vi "StateMachine V2.vi"() -> ()   [LabVIEW 2014]
uses:
  <vilib>/DAQmx/create/channels.llb/DAQmx Create Channel (AI-Voltage-Basic).vi
  <vilib>/DAQmx/configure/timing.llb/DAQmx Timing (Sample Clock).vi
  <vilib>/DAQmx/read.llb/DAQmx Read (Analog 1D Wfm NChan NSamp).vi
  <vilib>/Waveform/WDTOps.llb/WDT Index Channel DBL.vi
  <resource>/objmgr/daqmx.rc
panel:
  in  "Error In":errorcluster
  out "Final Data Array":dbl[][](array[numeric])
  in  "index":i32 caption="Index"
  out "Time & Y Array":dbl[][](array[numeric])
  out "Time Array":dbl[](array[numeric])
  out "Y Array":dbl[](array[numeric])
  out "Data Logging Done?":bool
  in  "Write Data in File":bool
  out "Recording ON time [ms]":u32
  out "Timer-Wert (ms)":u32
  in  "Timer [ms]":u32=2000
  out "Storing ON?":bool
  in  "Stopp":bool
  in  "Store Data in Array":bool
  out "State":T1(ring)
  out "Signalverlaufsgraph":waveform(dbl)[](graph)
  in  "samples per channel":i32=256 caption="Samples pro Kanal"
  out "SampleTakt.Rate":dbl
  in  "rate":dbl=2560.0 caption="Rate" format="%0.2f"
  in  "sample mode":i32(ring)=10123 caption="Sample-Modus" items=["Endliche Anzahl"=10178, "Kontinuierlich"=10123, "Einzelwert (HW-getaktet)"=12522]
  in  "physical channels":tag="Dev5/ai0" caption="Physikalische Kanäle"
  in  "maximum value":dbl=5.0 caption="Maximum" format="%0.2f"
  in  "minimum value":dbl=-5.0 caption="Minimum" format="%0.2f"
  in  "input terminal configuration":i32(ring)=-1 caption="Schaltung des Eingangsanschlusses" items=["Standard"=-1, "RSE"=10083, "NRSE"=10078, "Differentiell"=10106, "Pseudodifferentiell"=12529]
  # "Not currently useful"
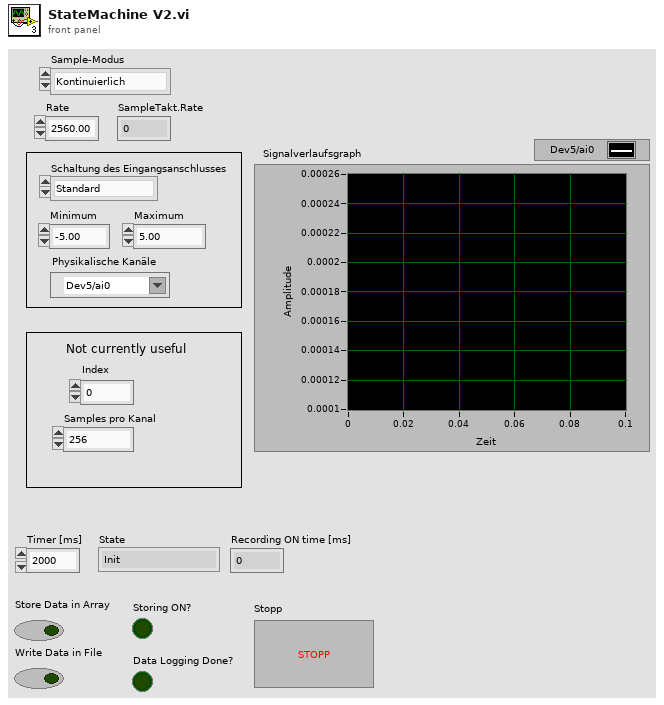
[diagram p1: front panel]
types:
  T1 = enum16{"Init", "Waiting for Trigger", "Storing Data in Array", "Log Data in File", "Shut Down"}
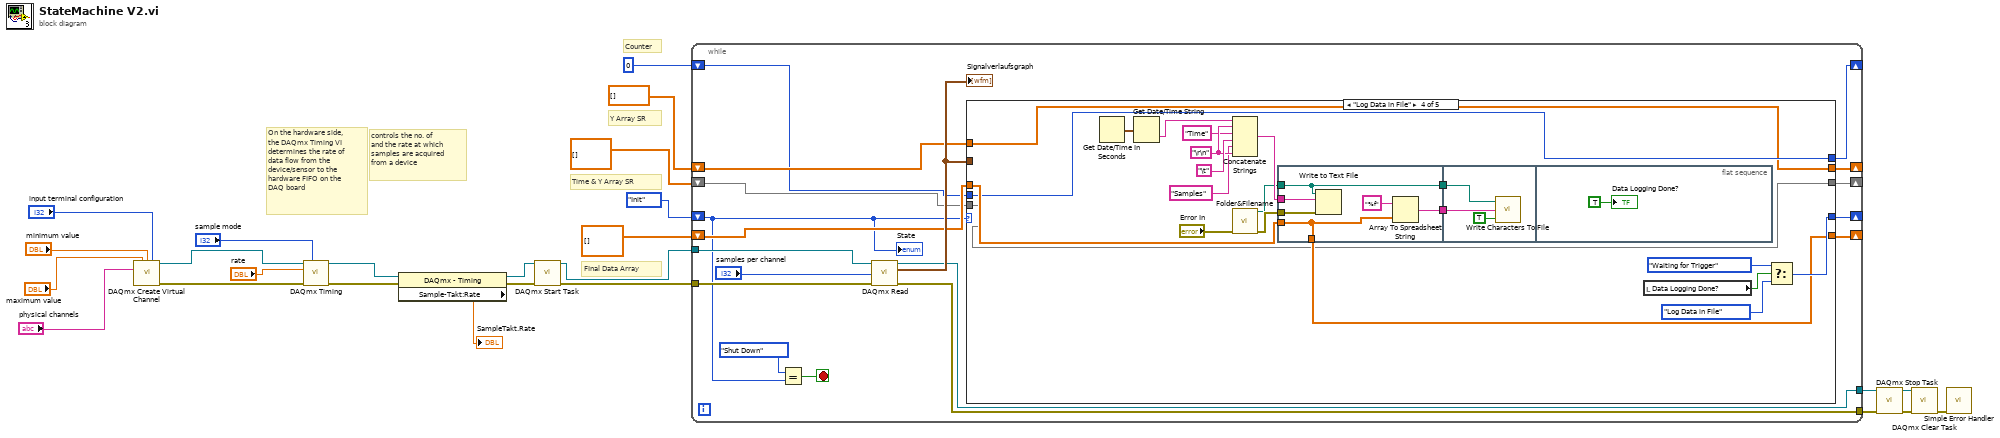
[diagram p0: block diagram]
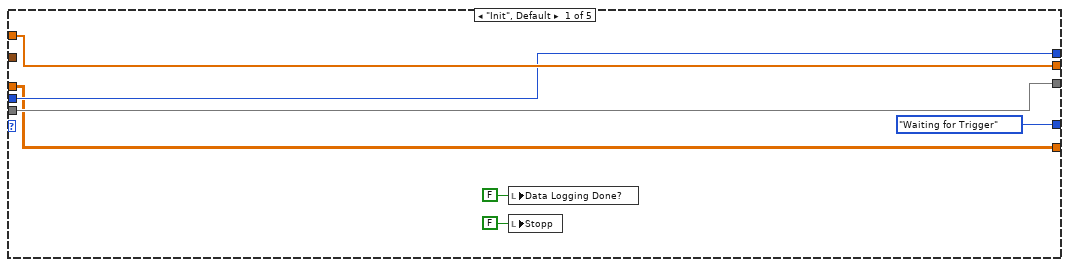
[diagram p2: hidden frame]
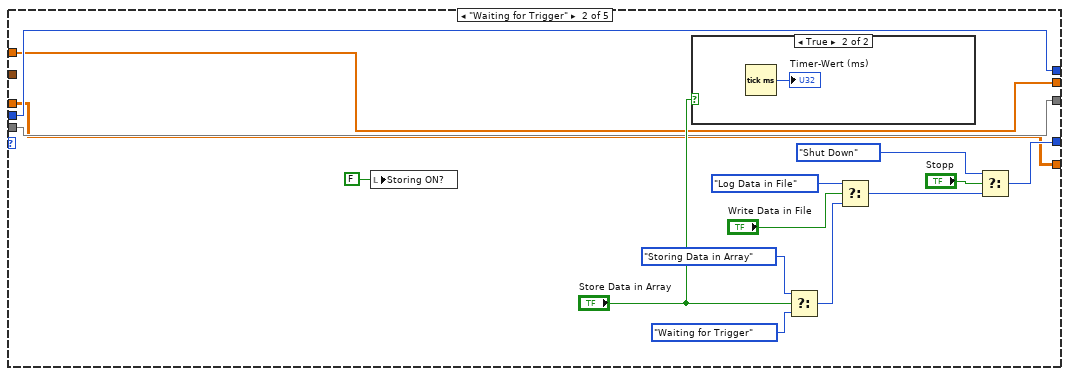
[diagram p3: hidden frame]
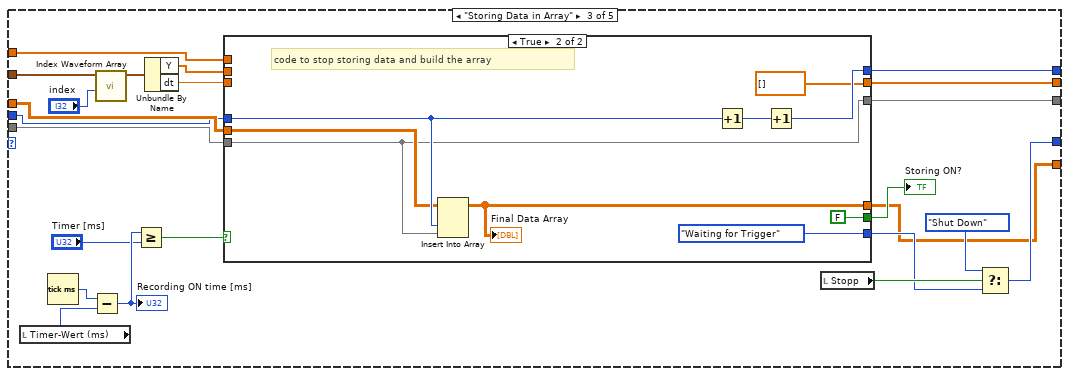
[diagram p5: hidden frame]
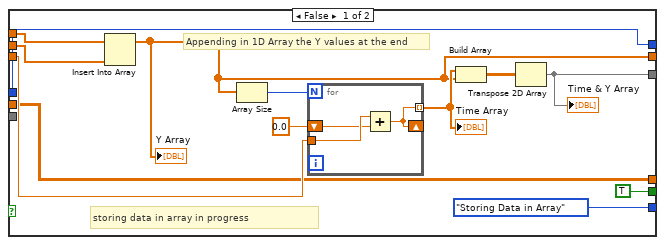
[diagram p6: hidden frame]
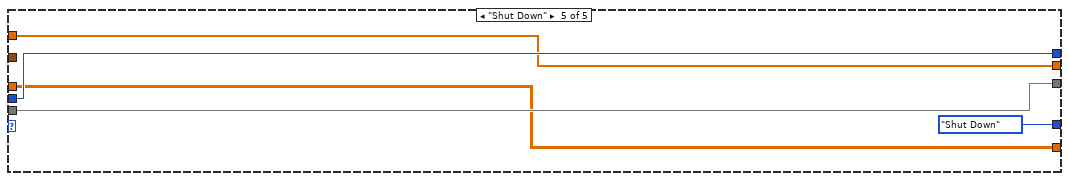
[diagram p7: hidden frame]
diagram:
  # "Counter"
  # "FInal Data Array"
  # "Time & Y Array SR"
  # "Y Array SR"
  # "controls the no. of \nand the rate at which \nsamples are acquired \nfrom a device"
  # "On the hardware side,\nthe DAQmx Timing VI\ndetermines the rate of \ndata flow from the \ndevice/sensor to the \nhardware FIFO on the \nDAQ board"
  n1 = call-poly <vilib>:"DAQmx Create Virtual Channel.vi"("maximum value"="maximum value", "minimum value"="minimum value", "input terminal configuration"="input terminal configuration", "physical channels"="physical channels") -> ("task out"=w21:refnum<k21>, "error out"=w20:errorcluster)  [unwired: 10 in]
  n2 = call-poly <vilib>:"DAQmx Timing.vi"("task/channels in"=w21, "sample mode"="sample mode", "rate"="rate", "error in"=w20) -> ("task out"=w17:refnum<k21>, "error out"=w16:errorcluster)  [unwired: 10 in]
  n3 = property class="DAQmx - Timing"(reference=w17, error in=w16) -> (reference out=w15:refnum<k21>, error out=w14:errorcluster, "Sample-Takt:Rate"=→"SampleTakt.Rate":dbl)
  n4 = call <vilib>:"DAQmx Start Task.vi"("task/channels in"=w15, "error in"=w14) -> ("task out"=w12:refnum<k21>, "error out"=w11:errorcluster)  [unwired: 12 in]
  n5 = while {
    tunnel: w12 -> [w42]
    tunnel: w11 -> [w41]
    shift-right: [w40] -> _
    shift-left: T1."Init" ("State") -> [w29]
    tunnel: [w28] -> w6
    tunnel: [w37] -> w5
    shift-right: [w35] -> _
    shift-left: dbl[] [] -> [w34]
    shift-right: [w33] -> _
    shift-left: dbl[][] [] -> [w32]
    shift-right: [w31] -> _
    shift-left: dbl[][] [] -> [w30]
    shift-right: [w27] -> _
    shift-left: i8 0 ("counter") -> [w26]
    stop <- w38 stop-if-true
    n6 = Equal?(x=T1."Shut Down" ("State"), y=w29) -> (x = y?=w38:bool)
    n7 = call-poly <vilib>:"DAQmx Read.vi"("task/channels in"=w42, "number of samples per channel"="samples per channel", "error in"=w41) -> ("task out"=w28:refnum<k21>, "data"=w36:waveform(dbl)[], "error out"=w37:errorcluster)  [unwired: 10 in]
    "Signalverlaufsgraph" <- w36
    n8 = case shown="\"Log Data in File\"" w29 {
      tunnel: [T1."Waiting for Trigger" ("State") w61 w80 w132 T1."Shut Down" ("State")] -> w40
      tunnel: w36 -> [_ _ w79 _ _]
      tunnel: [w46 w53 w74 w116 w146] -> w35
      tunnel: w34 -> [w46 w53 w73 w116 w146]
      tunnel: [w44 w51 w72 w119 w147] -> w33
      tunnel: w32 -> [w44 w51 w71 w118 w147]
      tunnel: [w47 w52 w70 w115 w149] -> w31
      tunnel: w30 -> [w47 w52 w69 w115 w149]
      tunnel: [w45 w54 w68 w117 w148] -> w27
      tunnel: w26 -> [w45 w54 w67 w117 w148]
      frame "Init", Default {
        n9 = local write "Data Logging Done?"(FALSE ("Data Logging Done?")) -> ()
        n10 = local write "Stopp"(FALSE ("Stopp")) -> ()
      }
      frame "Waiting for Trigger" {
        n11 = local write "Storing ON?"(FALSE ("Recording ON?")) -> ()
        n12 = case shown="True" "Store Data in Array" {
          frame False {
          }
          frame True {
            n13 = Tick Count (ms)() -> (millisecond timer value=→"Timer-Wert (ms)":u32)
          }
        }
        n14 = Select(t=T1."Storing Data in Array" ("State"), s="Store Data in Array", f=T1."Waiting for Trigger" ("State")) -> (s? t:f=w56:T1)
        n15 = Select(t=T1."Log Data in File" ("State"), s="Write Data in File", f=w56) -> (s? t:f=w55:T1)
        n16 = Select(t=T1."Shut Down" ("State"), s="Stopp", f=w55) -> (s? t:f=w61:T1)
      }
      frame "Storing Data in Array" {
        n17 = local read "Timer-Wert (ms)"() -> (w88:u32)
        n18 = Tick Count (ms)() -> (millisecond timer value=w89:u32)
        n19 = Subtract(x=w89, y=w88) -> (x-y=w87:u32)
        "Recording ON time [ms]" <- w87
        n20 = call-poly <vilib>:"Index Waveform Array.vi"("index"="index", "waveform array"=w79) -> ("waveform"=w77:waveform(dbl))  [unwired: 8 in, 1 out]
        n21 = Greater Or Equal?(x=w87, y="Timer [ms]") -> (x >= y?=w85:bool)
        n22 = Unbundle By Name(w77) -> ("Y"=w76:dbl[], "dt"=w75:dbl)
        n23 = case shown="True" w85 {
          tunnel: [TRUE FALSE] -> w84
          tunnel: [T1."Storing Data in Array" ("State") T1."Waiting for Trigger" ("State")] -> w81
          tunnel: w76 -> [w95 _]
          tunnel: w75 -> [w96 _]
          tunnel: [w92 dbl[] []] -> w74
          tunnel: w73 -> [w94 _]
          tunnel: [w91 w112] -> w72
          tunnel: w71 -> [w91 w108]
          tunnel: [w93 w107] -> w70
          tunnel: w69 -> [_ w107]
          tunnel: [w90 w110] -> w68
          tunnel: w67 -> [w90 w109]
          frame False {
            # "Appending in 1D Array the Y values at the end"
            # "storing data in array in progress"
            n24 = Insert Into Array(array=w94, new element=w95) -> (w92:dbl[])  [unwired: 1 in]
            "Y Array" <- w92
            n25 = Array Size(array=w92) -> (size(s)=w97:i32)
            n26 = for {
              N: w97 -> [_]
              tunnel: w96 -> [w105]
              shift-right: [w103] -> _
              shift-left: 0.0 -> [w104]
              tunnel: [w103] -> w98 mode=indexing
              n27 = Add(x=w105, y=w104) -> (x+y=w103:dbl)
            }
            "Time Array" <- w98
            n28 = Build Array(w98, w92) -> (w99:dbl[][])
            n29 = Transpose 2D Array(2D array=w99) -> (transposed array=w93:dbl[][])
            "Time & Y Array" <- w93
          }
          frame True {
            # "code to stop storing data and build the array"
            n30 = Insert Into Array(array=w108, index (col)=w109, new element=w107) -> (w112:dbl[][])  [unwired: 1 in]
            "Final Data Array" <- w112
            n31 = Increment(x=w109) -> (x+1=w111:i8)
            n32 = Increment(x=w111) -> (x+1=w110:i8)
          }
        }
        "Storing ON?" <- w84
        n33 = local read "Stopp"() -> (w83:bool)
        n34 = Select(t=T1."Shut Down" ("State"), s=w83, f=w81) -> (s? t:f=w80:T1)
      }
      frame "Log Data in File" {
        w129 = "\r\n" ("String")
        n35 = Get Date/Time In Seconds() -> (seconds since 1Jan1904=w130:timestamp)
        n36 = Get Date/Time String(seconds (now)=w130) -> (time string=w128:string)  [unwired: 2 in, 1 out]
        n37 = Concatenate Strings(w128, w129, "Time" ("Header 1"), "\t", "Samples" ("Header 2"), w129) -> (w124:string)
        n38 = call "Folder&Filename.vi"("Fehler (Eingang, kein Fehler)"="Error In") -> ("Hinzugefügter Pfad"=w122:path, "Fehler (Ausgang)"=w123:errorcluster)  [unwired: 13 in]
        n39 = flat-sequence {
          tunnel: w124 -> [w140]
          tunnel: w123 -> [w139]
          tunnel: w122 -> [w138]
          tunnel: w118 -> [w136]
          tunnel: [w138] -> w121
          tunnel: [w137] -> w120
          tunnel: [w136] -> w119
          tunnel: w121 -> [w142]
          tunnel: w120 -> [w143]
          frame #0 {
            n40 = Write to Text File(file (use dialog)=w138, text=w140, error in=w139) -> ()  [unwired: 1 in, 3 out]
            n41 = Array To Spreadsheet String(array=w136, 3:"%f" ("Format-String")) -> (spreadsheet string=w137:string)  [unwired: 1 in]
          }
          frame #1 {
            n42 = call <vilib>:"Write Characters To File.vi"("append to file? (new file:F)"=TRUE, "character string"=w143, "file path (dialog if empty)"=w142) -> ()  [unwired: 2 in, 1 out]
          }
          frame #2 {
            "Data Logging Done?" <- TRUE ("Data Logging Done?")
          }
        }
        n43 = local read "Data Logging Done?"() -> (w135:bool)
        n44 = Select(t=T1."Waiting for Trigger" ("State"), s=w135, f=T1."Log Data in File" ("State")) -> (s? t:f=w132:T1)
      }
      frame "Shut Down" {
      }
    }
    "State" <- w29
  }
  n45 = call <vilib>:"DAQmx Stop Task.vi"("task/channels in"=w6, "error in"=w5) -> ("task out"=w8:refnum<k21>, "error out"=w7:errorcluster)  [unwired: 12 in]
  n46 = call <vilib>:"DAQmx Clear Task.vi"("task in"=w8, "error in"=w7) -> ("error out"=w9:errorcluster)  [unwired: 13 in]
  n47 = call <vilib>:"Simple Error Handler.vi"("error in (no error)"=w9) -> ()  [unwired: 4 in, 5 out]
